vi "ConvertReadRegisterToString.vi"(11 "Register":T1) -> (3 "Register":string)   [LabVIEW 2013, in "Keithley-2602.lvlib"]
uses:
  Keithley-2602.lvlib
  Public/Controls/Register.ctl
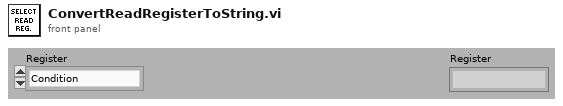
[diagram p1: front panel]
types:
  T1 = typedef "Keithley-2602.lvlib/Register.ctl" = enum16{"Condition", "Event", "Enable", "Positive Transition", "Negative Transition"}
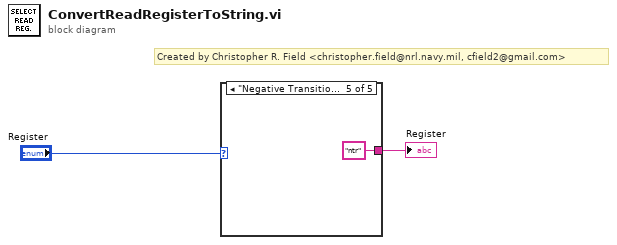
[diagram p0: block diagram]
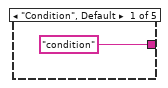
[diagram p2: hidden frame]
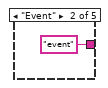
[diagram p3: hidden frame]
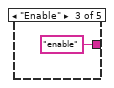
[diagram p4: hidden frame]
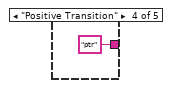
[diagram p5: hidden frame]
diagram:
  # "Created by Christopher R. Field <christopher.field@nrl.navy.mil, cfield2@gmail.com>"
  n1 = case shown="\"Negative Transition\"" "Register" {
    tunnel: ["condition" "event" "enable" "ptr" "ntr"] -> w2
    frame "Condition", Default {
    }
    frame "Event" {
    }
    frame "Enable" {
    }
    frame "Positive Transition" {
    }
    frame "Negative Transition" {
    }
  }
  "Register" <- w2
